vi "Generate Clothoid Trajectory.vi"(4 "Angular Limits":T4={"Velocity (deg/s)"=6.0, "Accel (deg/s^2)"=15.0, "Jerk (deg/s^3)"=150.0} {"Jerk (deg/s^3)" min=0.0 step=1.0; "Accel (deg/s^2)" min=0.0; "Velocity (deg/s)" min=0.0}, 5 "Drive Type":T3=enum."Holonomic", 6 "Overrides":T5 {"Angle Override" step=5.0; "Velocity Override" step=5.0; "Angular Override" step=5.0}, 7 "Stoopid Overlap %":dbl min=0.0, 8 "Conditions":T7, 9 "Limits":T6={"Velocity (fps)"=6.0, "Accel (fps^2)"=15.0, "Jerk (fps^3)"=150.0, "StoopidFast (fps)"=6.0} {"StoopidFast (fps)" min=0.0; "Jerk (fps^3)" min=0.0 step=1.0; "Accel (fps^2)" min=0.0; "Velocity (fps)" min=0.0}, 10 "Sample Period (s)":dbl=0.02, 11 "WayPoints":cluster{"x":dbl, "y":dbl, "th":dbl}[](array[cluster])) -> (0 "Updated Waypoints":cluster{"x":dbl, "y":dbl, "th":dbl}[](array[cluster]), 1 "Valid":bool, 2 "Time & Dist":cluster{"Time (s)":dbl, "Distance (ft)":dbl}, 3 "Trajectory Data Out":T2(array[cluster]))   [LabVIEW 2025]
uses:
  Types/Limits.ctl
  Types/Overrides.ctl
  Types/Angluar Limits.ctl
  Types/Drive Type.ctl
  Types/Segment Type.ctl
  Types/Speeds.ctl
panel:
  out "Distance (ft)":dbl
  out "Time (s)":dbl
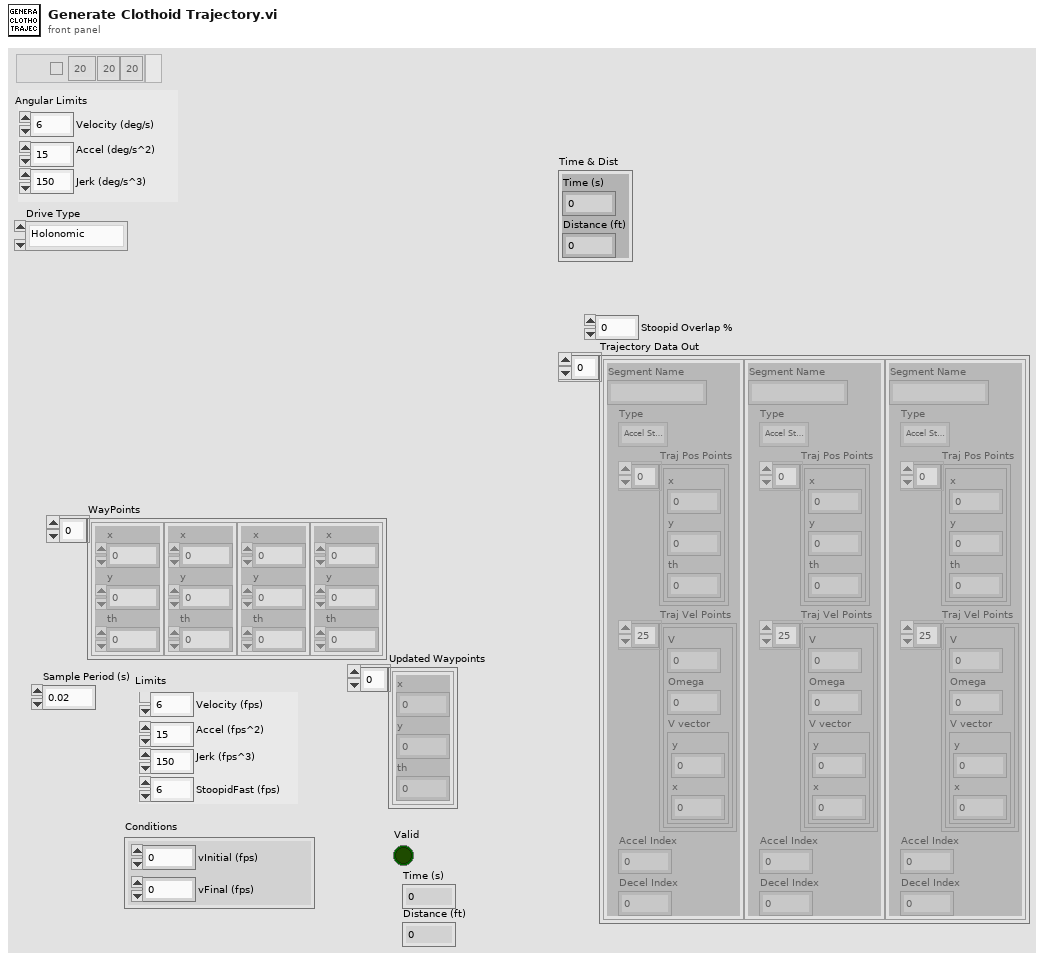
[diagram p1: front panel]
types:
  T1 = typedef "Segment Type.ctl" = enum16{"Accel Straight", "Const Straight", "Blend", "Circle", "Bezier"}
  T2 = cluster{"Segment Name":string, "Type":T1, "Traj Pos Points":cluster{"x":dbl, "y":dbl, "th":dbl}[], "Traj Vel Points":cluster{"V":dbl, "Omega":dbl, "V vector":cluster{"y":dbl, "x":dbl}}[], "Accel Index":i32, "Decel Index":i32}[]
  T3 = typedef "Drive Type.ctl" = enum16{"Nonholonomic", "Holonomic"}
  T4 = typedef "Angluar Limits.ctl" = cluster{"Velocity (deg/s)":dbl, "Accel (deg/s^2)":dbl, "Jerk (deg/s^3)":dbl}
  T5 = typedef "Overrides.ctl" = cluster{"Count":string, "Angular Override":dbl, "Enabled?":bool, "Velocity Override":dbl, "Angle Override":dbl}[]
  T6 = typedef "Limits.ctl" = cluster{"Velocity (fps)":dbl, "Accel (fps^2)":dbl, "Jerk (fps^3)":dbl, "StoopidFast (fps)":dbl}
  T7 = cluster{"vInitial (fps)":dbl, "vFinal (fps)":dbl}
  T8 = typedef "Speeds.ctl" = cluster{"maxV (fps)":dbl, "Accel Limit (fps^2)":dbl, "Initial V (fps)":dbl, "Sample Period (s)":dbl, "Jerk Limit (fps^3)":dbl, "Distances":cluster{"distance (ft)":dbl, "baseline (ft)":dbl, "high (ft)":dbl}[]}
  T9 = cluster{"Count":string, "Angular Override":dbl, "Enabled?":bool, "Velocity Override":dbl, "Angle Override":dbl}
  T10 = cluster{"Point Out":cluster{"x":dbl, "y":dbl, "th":dbl}, "Point Out":cluster{"x":dbl, "y":dbl, "th":dbl}, "Valid":bool}[]
  T11 = typedef "BlendType.ctl" = cluster{"Scaling":dbl, "Length":dbl, "Angle":dbl, "Vertex Dist":dbl, "ParaTime":dbl, "ExtraArc":dbl, "Center Point":cluster{dbl, dbl}, "Radius":dbl}
  T12 = cluster{"Segment Name":string, "Type":enum16{"Accel Straight", "Const Straight", "Blend", "Circle"}, "Traj Pos Points":cluster{"x":dbl, "y":dbl, "th":dbl}[], "Traj Vel Points":cluster{"V":dbl, "th":dbl}[], "Accel Index":i32, "Decel Index":i32}
  T13 = cluster{"Segment Name":string, "Type":enum16{"Accel Straight", "Const Straight", "Blend", "Circle"}, "Traj Pos Points":cluster{"x":dbl, "y":dbl, "th":dbl}[], "Traj Vel Points":cluster{"V":dbl, "th":dbl}[], "Accel Index":i32, "Decel Index":i32}[]
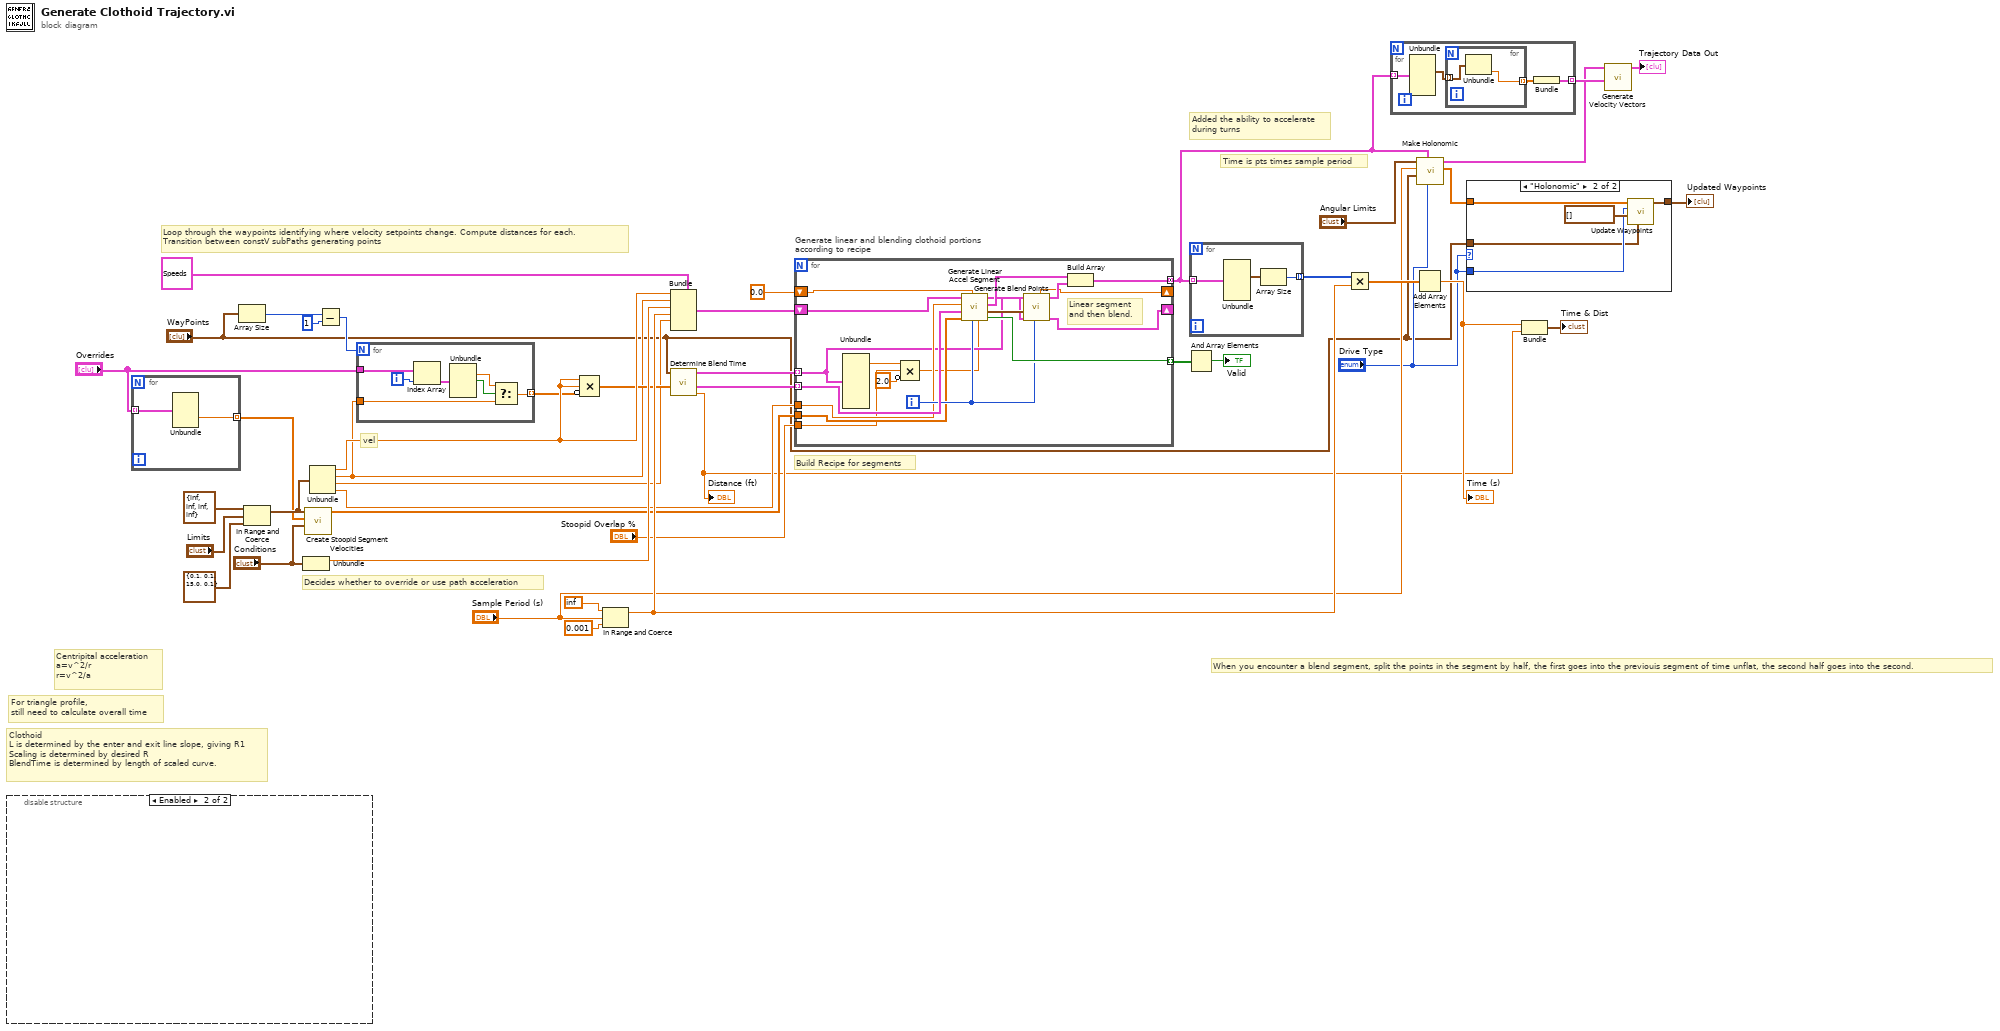
[diagram p0: block diagram]
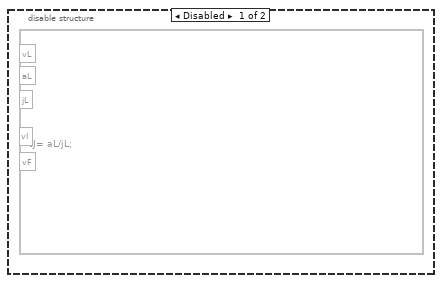
[diagram p3: hidden frame]
diagram:
  # "When you encounter a blend segment, split the points in the segment by half, the first goes into the previouis segment of time unflat, the second half goes into the second."
  # "Loop through the waypoints identifying where velocity setpoints change. Compute distances for each.\nTransition between constV subPaths generating points"
  # "Added the ability to accelerate\nduring turns"
  # "Decides whether to override or use path acceleration"
  # "For triangle profile,\nstill need to calculate overall time"
  # "Build Recipe for segments"
  # "Time is pts times sample period"
  # "Clothoid\nL is determined by the enter and exit line slope, giving R1\nScaling is determined by desired R\nBlendTime is determined by length of scaled curve."
  # "Centripital acceleration\na=v^2/r\nr=v^2/a"
  # "vel"
  n1 = disable-structure shown="Enabled" {
    frame Disabled {
      n2 = formula code="tJ= aL/jL;"() -> ()  [unwired: 5 in]
    }
    frame Enabled {
    }
  }
  n3 = for {
    tunnel: "Overrides" -> [w45] mode=indexing
    tunnel: [w46] -> w18 mode=indexing
    n4 = Unbundle(w45) -> ("Velocity Override"=w46:dbl)  [unwired: 4 out]
  }
  n5 = Array Size(array="WayPoints") -> (size(s)=w20:i32)
  n6 = In Range and Coerce(upper limit=T6 {"Velocity (fps)"=inf, "Accel (fps^2)"=inf, "Jerk (fps^3)"=inf, "StoopidFast (fps)"=inf} ("Limits"), x="Limits", lower limit=T6 {"Velocity (fps)"=0.1, "Accel (fps^2)"=0.1, "Jerk (fps^3)"=15.0, "StoopidFast (fps)"=0.1} ("Limits")) -> (coerced(x)=w28:T6)  [unwired: 1 out]
  n7 = Unbundle("Conditions") -> ("vInitial (fps)"=w34:dbl)  [unwired: 1 out]
  n8 = call "Create Stoopid Segment Velocities.vi"("Conditions"="Conditions", "Velocities"=w18, "Limits"=w28) -> ("Velocities"=w27:dbl[])  [unwired: 8 in]
  n9 = Unbundle(w28) -> ("Velocity (fps)"=w33:dbl, "Accel (fps^2)"=w15:dbl, "Jerk (fps^3)"=w16:dbl, "StoopidFast (fps)"=w17:dbl)
  n10 = Subtract(x=w20, y=1) -> (x-y=w21:i32)
  n11 = for {
    N: w21 -> [_]
    tunnel: "Overrides" -> [w53]
    tunnel: w15 -> [w50]
    tunnel: [w49] -> w22 mode=indexing
    i -> [w47]
    n12 = Index Array(array=w53, index=w47) -> (element=w48:T9)
    n13 = Unbundle(w48) -> ("Angular Override"=w51:dbl, "Enabled?"=w52:bool)  [unwired: 3 out]
    n14 = Select(t=w51, s=w52, f=w50) -> (s? t:f=w49:dbl)
  }
  n15 = Compound Arithmetic op=MULTIPLY(w33, w33, invert w22) -> (w32:dbl[])
  n16 = In Range and Coerce(upper limit=inf, x="Sample Period (s)", lower limit=0.001) -> (coerced(x)=w36:dbl)  [unwired: 1 out]
  n17 = Bundle(cluster=T8 {"maxV (fps)"=6.0, "Accel Limit (fps^2)"=15.0, "Initial V (fps)"=5.999999999999998, "Sample Period (s)"=0.02, "Jerk Limit (fps^3)"=150.0, "Distances"=[{"distance (ft)"=0.0, "baseline (ft)"=0.0, "high (ft)"=0.0}, {"distance (ft)"=0.3647338133499236, "baseline (ft)"=1.8397338133499224, "high (ft)"=0.9397338133499229}]} ("Speeds in"), "maxV (fps)"=w33, "Accel Limit (fps^2)"=w15, "Initial V (fps)"=w34, "Sample Period (s)"=w36, "Jerk Limit (fps^3)"=w16) -> (w26:T8)  [unwired: 1 in]
  n18 = call "Determine Blend Time.vi"("Min R"=w32, "WayPoints"="WayPoints") -> ("Distance"=w13:dbl, "Linear Info"=w43:T10, "Blends"=w42:T11[])  [unwired: 6 in, 1 out]
  "Distance (ft)" <- w13
  n19 = for "Generate linear and blending clothoid portions\naccording to recipe" {
    tunnel: [w72] -> w4 mode=concatenating
    tunnel: w42 -> [w58] mode=indexing
    shift-right: [w71] -> _
    shift-left: w26 -> [w60]
    tunnel: w43 -> [w66] mode=indexing
    tunnel: [w65] -> w39 mode=indexing
    shift-right: [w64] -> _
    shift-left: 0.0 ("Final Acceleration") -> [w63]
    tunnel: w27 -> [w61]
    tunnel: w17 -> [w59]
    tunnel: "Stoopid Overlap %" -> [w56]
    i -> [w62]
    # "Linear segment\nand then blend."
    n20 = Unbundle(w58) -> ("Length"=w57:dbl)  [unwired: 7 out]
    n21 = Compound Arithmetic op=MULTIPLY(w57, w56, invert 2.0 ("value")) -> (w54:dbl)
    n22 = call "Generate Linear Accel Segment.vi"("Stoopid Overlap distance"=w54, "Index"=w62, "Initial Acceleration"=w63, "Velocities"=w61, "Linear Info"=w66, "Stoopid V"=w59, "Speeds in"=w60) -> ("Valid"=w65:bool, "Final Position"=w70:cluster{dbl, dbl, dbl}, "Trajectory Segment"=w68:T12, "Speeds out"=w67:T8)  [unwired: 1 out]
    n23 = call "Generate Blend Points.vi"("Index"=w62, "Speeds in"=w67, "Initial Point"=w70, "Blend Info"=w58) -> ("Speeds out"=w71:T8, "Trajectory Segment"=w69:T12, "Final Acceleration"=w64:dbl)  [unwired: 5 in]
    n24 = Build Array(w68, w69) -> (w72:T13)
  }
  n25 = And Array Elements(Boolean array=w39) -> (logical AND=→"Valid":bool)
  n26 = for {
    tunnel: w4 -> [w75] mode=indexing
    tunnel: [w74] -> w41 mode=indexing
    n27 = Unbundle(w75) -> ("Traj Pos Points"=w73:cluster{"x":dbl, "y":dbl, "th":dbl}[])  [unwired: 5 out]
    n28 = Array Size(array=w73) -> (size(s)=w74:i32)
  }
  n29 = Multiply(x=w41, y=w36) -> (x*y=w40:dbl[])
  n30 = for {
    tunnel: w4 -> [w79] mode=indexing
    tunnel: [w77] -> w3 mode=indexing
    n31 = Unbundle(w79) -> ("Traj Pos Points"=w76:cluster{"x":dbl, "y":dbl, "th":dbl}[])  [unwired: 5 out]
    n32 = for {
      tunnel: [w80] -> w78 mode=indexing
      tunnel: w76 -> [w81] mode=indexing
      n33 = Unbundle(w81) -> ("th"=w80:dbl)  [unwired: 2 out]
    }
    n34 = Bundle(w78) -> (w77:cluster{dbl[]})  [unwired: 1 in]
  }
  n35 = Add Array Elements(numeric array=w40) -> (sum=w14:dbl)
  "Time (s)" <- w14
  n36 = call "Make Holonomic.vi"("Drive Type"="Drive Type", "Trajectory Data In"=w4, "WayPoints"="WayPoints", "Sample Period (s)"="Sample Period (s)", "Angular Limits"="Angular Limits") -> ("Headings"=w10:dbl[], "Trajectory Data Out"=w2:T13)  [unwired: 5 in]
  n37 = case shown="\"Holonomic\"" "Drive Type" {
    tunnel: "Drive Type" -> [_ w86]
    tunnel: w10 -> [_ w85]
    tunnel: [w82 w84] -> w5
    tunnel: "WayPoints" -> [w82 w83]
    frame "Nonholonomic", Default {
    }
    frame "Holonomic" {
      n38 = call "Update Waypoints.vi"("Waypoints"=w83, "Tangents"=cluster{sgl, sgl}[] [], "Drive Type"=w86, "X"=w85) -> ("Updated Waypoints"=w84:cluster{"x":dbl, "y":dbl, "th":dbl}[])  [unwired: 7 in]
    }
  }
  "Updated Waypoints" <- w5
  n39 = Bundle(w14, "Distance"=w13) -> (→"Time & Dist":cluster{dbl, "Distance":dbl})  [unwired: 1 in]
  n40 = call "Generate Velocity Vectors.vi"("Nonholonomic Headings"=w3, "Trajectory Data In"=w2) -> ("Trajectory Data Out"=→"Trajectory Data Out":T2)  [unwired: 9 in]
